vi "uTTA_ucf_ReadChannelCal.vi"(7 "Section":string, 8 "error in":errorcluster, 11 "Refnum in":T2) -> (0 "error out":errorcluster, 1 "QuadGain":dbl, 2 "Cal Status":T1, 3 "Refnum out":T2, 4 "Offset":dbl, 6 "LinGain":dbl)   [LabVIEW 2021]
uses:
  <vilib>/Utility/config.llb/Config Data RefNum.ctl
  uTTA_Device_Driver/uTTA_Controls/CTL_uTTA_TSP_CalStatus.ctl
  <vilib>/Utility/config.llb/Read Key (String).vi
  <vilib>/Utility/config.llb/Read Key (U32).vi
  <vilib>/Utility/config.llb/NI_LVConfig.lvlib
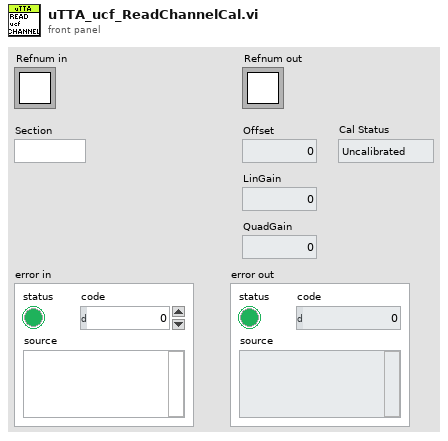
[diagram p1: front panel]
types:
  T1 = typedef "CTL_uTTA_TSP_CalStatus.ctl" = enum16{"Uncalibrated", "Calibrated", "Dummy"}
  T2 = typedef "NI_LVConfig.lvlib/Config Data RefNum.ctl" = refnum<k1>
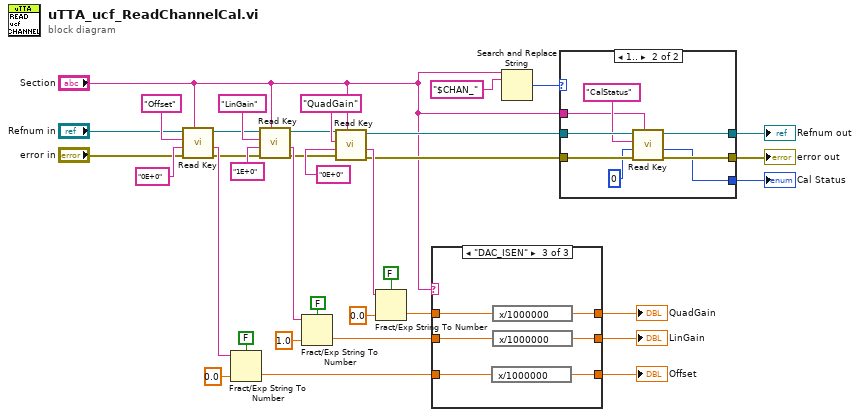
[diagram p0: block diagram]
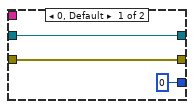
[diagram p2: hidden frame]
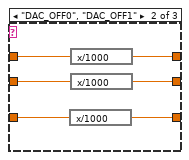
[diagram p4: hidden frame]
diagram:
  n1 = call-poly <vilib>:"Read Key.vi"("section"="Section", "error in (no error)"="error in", "default value"="0E+0", "key"="Offset", "refnum"="Refnum in") -> ("error out"=w18:errorcluster, "value"=w27:string, "refnum out"=w17:T2)  [unwired: 3 in, 1 out]
  n2 = Fract/Exp String To Number(use system decimal point (T)=FALSE, string=w27, default (0 dbl)=0.0 ("default (0 DBL)")) -> (number=w10:dbl)  [unwired: 1 in, 1 out]
  n3 = call-poly <vilib>:"Read Key.vi"("section"="Section", "error in (no error)"=w18, "default value"="1E+0", "key"="LinGain", "refnum"=w17) -> ("error out"=w19:errorcluster, "value"=w31:string, "refnum out"=w20:T2)  [unwired: 3 in, 1 out]
  n4 = Fract/Exp String To Number(use system decimal point (T)=FALSE, string=w31, default (0 dbl)=1.0 ("default (0 DBL)")) -> (number=w12:dbl)  [unwired: 1 in, 1 out]
  n5 = call-poly <vilib>:"Read Key.vi"("section"="Section", "error in (no error)"=w19, "default value"="0E+0", "key"="QuadGain", "refnum"=w20) -> ("error out"=w4:errorcluster, "value"=w35:string, "refnum out"=w5:T2)  [unwired: 3 in, 1 out]
  n6 = Fract/Exp String To Number(use system decimal point (T)=FALSE, string=w35, default (0 dbl)=0.0 ("default (0 DBL)")) -> (number=w14:dbl)  [unwired: 1 in, 1 out]
  n7 = case shown="\"DAC_ISEN\"" "Section" {
    tunnel: w14 -> [w38 w42 w48]
    tunnel: w12 -> [w37 w41 w47]
    tunnel: w10 -> [w36 w44 w50]
    tunnel: [w38 w39 w45] -> w13
    tunnel: [w37 w40 w46] -> w11
    tunnel: [w36 w43 w49] -> w9
    frame Default {
    }
    frame "DAC_OFF0", "DAC_OFF1" {
      n8 = expression code="x/1000"(w44) -> (w43:dbl)
      n9 = expression code="x/1000"(w42) -> (w39:dbl)
      n10 = expression code="x/1000"(w41) -> (w40:dbl)
    }
    frame "DAC_ISEN" {
      n11 = expression code="x/1000000"(w50) -> (w49:dbl)
      n12 = expression code="x/1000000"(w48) -> (w45:dbl)
      n13 = expression code="x/1000000"(w47) -> (w46:dbl)
    }
  }
  "Offset" <- w9
  "LinGain" <- w11
  "QuadGain" <- w13
  n14 = Search and Replace String(input string="Section", search string="$CHAN_") -> (number of replacements=w7:i32)  [unwired: 6 in, 3 out]
  n15 = case shown="1.." w7 {
    tunnel: w5 -> [w53 w61]
    tunnel: w4 -> [w52 w60]
    tunnel: [w53 w59] -> w3
    tunnel: [w52 w58] -> w2
    tunnel: "Section" -> [_ w54]
    tunnel: [u32 0 ("value") w57] -> w6
    frame 0, Default {
    }
    frame 1.. {
      n16 = call-poly <vilib>:"Read Key.vi"("section"=w54, "error in (no error)"=w60, "default value"=u32 0, "key"="CalStatus", "refnum"=w61) -> ("error out"=w58:errorcluster, "value"=w57:u32, "refnum out"=w59:T2)  [unwired: 3 in, 1 out]
    }
  }
  "error out" <- w2
  "Refnum out" <- w3
  "Cal Status" <- w6
